vi "Prepare Cargo Details.vi"(2 "Stacks Drawing":string[](array[string]), 3 "#Stacks":i32) -> (0 "Cargo":T1)   [LabVIEW 2020, in "AoC 2022.lvlib"]
uses:
  AoC 2022.lvlib
  Cargo.ctl
  <vilib>/Utility/miscctls.llb/LVMapReplaceAction.ctl
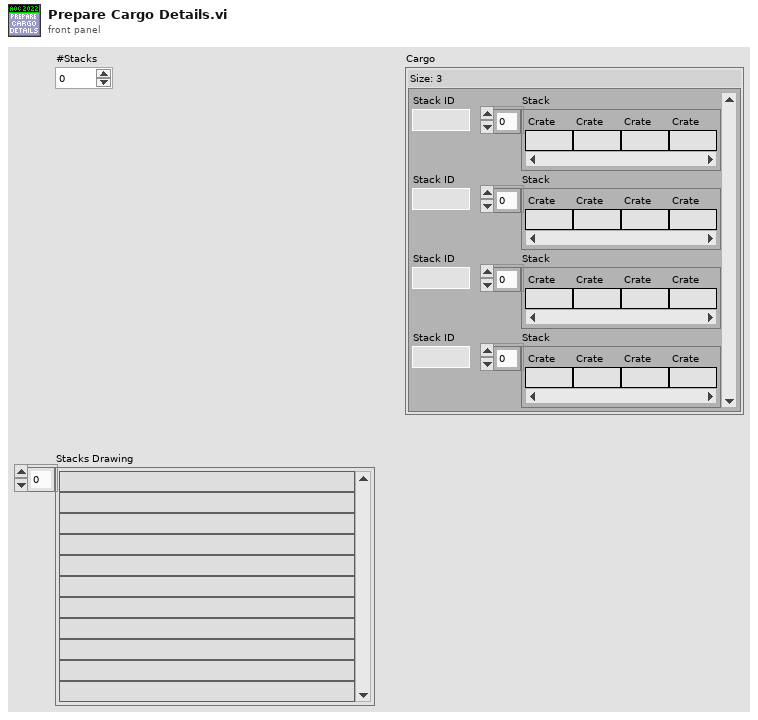
[diagram p1: front panel]
types:
  T1 = typedef "AoC 2022.lvlib/Cargo.ctl" = map{i32, string[]}
  T2 = typedef "LVMapReplaceAction.ctl" = enum32{"Modify Entry only if found", "Add or Modify Entry", "Delete Entry"}
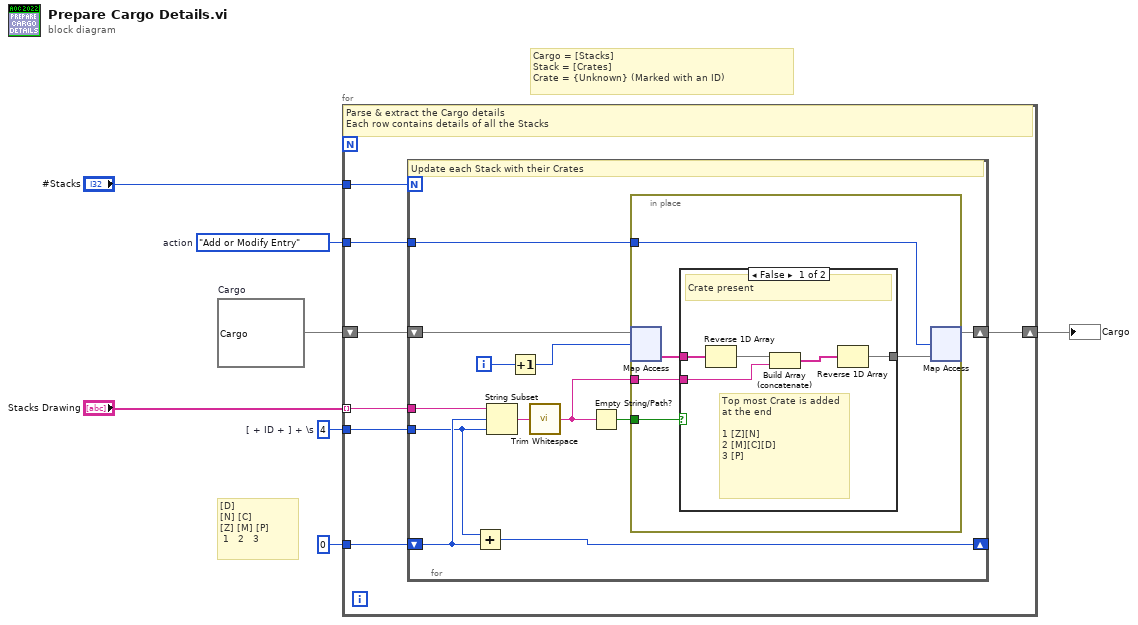
[diagram p0: block diagram]
diagram:
  w6 = LVMapReplaceAction."Add or Modify Entry"  # action
  w5 = T1 {}  # Cargo
  w3 = 4  # [ + ID + ] + \s
  # "[D]    \n[N] [C]    \n[Z] [M] [P]\n 1   2   3"
  # "Cargo = [Stacks]\nStack = [Crates]\nCrate = {Unknown} (Marked with an ID)"
  n1 = for {
    tunnel: "Stacks Drawing" -> [w14] mode=indexing
    tunnel: 0 -> [w13]
    tunnel: w3 -> [w12]
    tunnel: "#Stacks" -> [w11]
    shift-right: [w9] -> w7
    shift-left: w5 -> [w10]
    tunnel: w6 -> [w8]
    # "Parse & extract the Cargo details\nEach row contains details of all the Stacks"
    n2 = for {
      N: w11 -> [_]
      tunnel: w14 -> [w26]
      tunnel: w12 -> [w24]
      shift-right: [w23] -> _
      shift-left: w13 -> [w25]
      shift-right: [w20] -> w9
      shift-left: w10 -> [w22]
      tunnel: w8 -> [w19]
      i -> [w21]
      # "Update each Stack with their Crates"
      n3 = Add(x=w24, y=w25) -> (x+y=w23:i32)
      n4 = String Subset(string=w26, offset (0)=w25, length (rest)=w24) -> (substring=w18:string)
      n5 = Increment(x=w21) -> (x+1=w16:i32)
      n6 = call <vilib>:"Trim Whitespace.vi"("string"=w18) -> ("trimmed string"=w15:string)  [unwired: 1 in]
      n7 = Empty String/Path?(string/path=w15) -> (empty?=w17:bool)
      n8 = in-place {
        in-place-border: w19 -> [w31]
        in-place-border: w15 -> [w28]
        in-place-border: w17 -> [w27]
        n9 = in-place-map #1(w22, w16) -> (w30:string[])  [unwired: 1 in, 1 out]
        n10 = case shown="False" w27 {
          tunnel: w30 -> [w35 w37]
          tunnel: [w32 w37] -> w29
          tunnel: w28 -> [w36 _]
          frame False {
            # "Top most Crate is added at the end\n\n1 [Z][N]\n2 [M][C][D]\n3 [P]"
            # "Crate present"
            n11 = Reverse 1D Array(array=w35) -> (reversed array=w34:string[])
            n12 = Build Array (concatenate)(w34, w36) -> (w33:string[])
            n13 = Reverse 1D Array(array=w33) -> (reversed array=w32:string[])
          }
          frame True {
            # "Crate not present"
          }
        }
        n14 = in-place-map #1(w29, w31) -> (w20:T1)  [unwired: 2 out]
      }
    }
  }
  "Cargo" <- w7
